vi "Read States.vi"(8 "error in (no error)":errorcluster, 11 "PenaltyAttackerTactic in":refnum<class "PenaltyAttackerTactic.lvclass">) -> (0 "error out":errorcluster, 2 "States":enum16{"Exit", "Penalty"}(ring), 3 "PenaltyAttackerTactic out":refnum<class "PenaltyAttackerTactic.lvclass">)   [LabVIEW 2023, in "PenaltyAttackerTactic.lvclass"]
uses:
  PenaltyAttackerTactic.lvclass
  PenaltyAttackerTactic.lvclass/PenaltyAttackerTactic.ctl
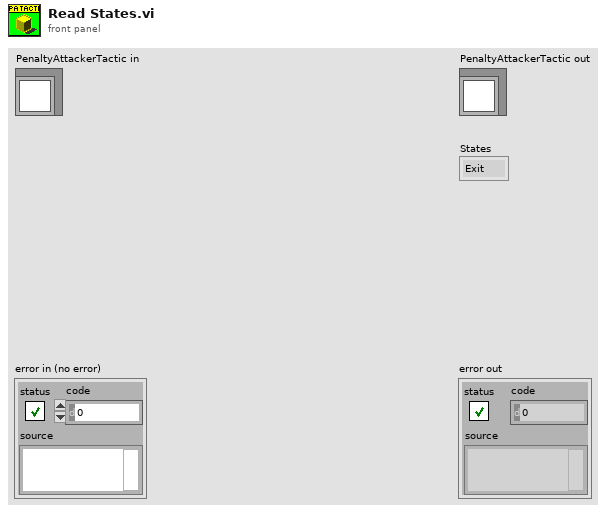
[diagram p1: front panel]
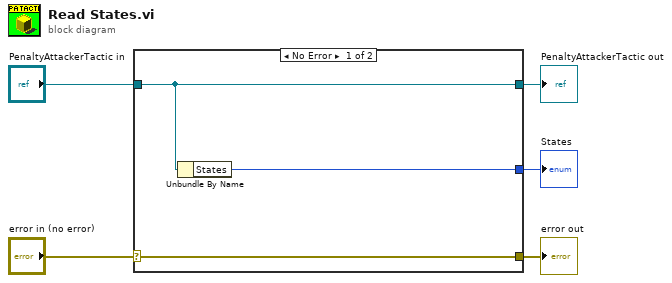
[diagram p0: block diagram]
diagram:
  n1 = case shown="No Error" "error in (no error)" {
    selector: "error in (no error)" -> [w8 w9]
    tunnel: [w8 w9] -> w4
    tunnel: [w7 w10] -> w2
    tunnel: "PenaltyAttackerTactic in" -> [w7 w10]
    tunnel: [w6 _] -> w1
    frame No Error {
      n2 = Unbundle By Name(w7) -> ("States"=w6:enum16{"Exit", "Penalty"})
    }
    frame Error {
    }
  }
  "error out" <- w4
  "PenaltyAttackerTactic out" <- w2
  "States" <- w1
